vi "Dequeue.vi"() -> ()   [LabVIEW 2019]
panel:
  out "Cliente":string
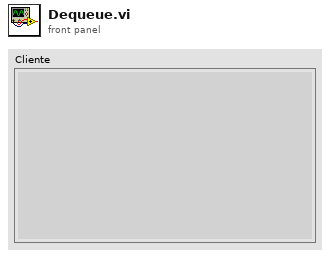
[diagram p1: front panel]
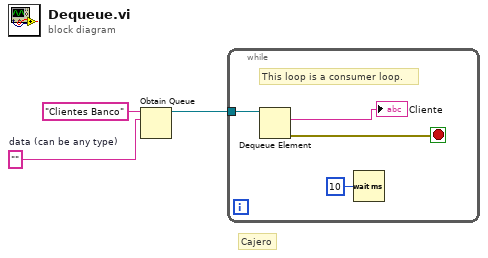
[diagram p0: block diagram]
diagram:
  w3 = ""  # data (can be any type)
  # "Cajero"
  n1 = Obtain Queue(name (unnamed)="Clientes Banco", element data type=w3) -> (queue out=w1:refnum<queue>)  [unwired: 3 in, 2 out]
  n2 = while {
    tunnel: w1 -> [w5]
    stop <- w7 stop-if-true
    # "This loop is a consumer loop."
    n3 = Dequeue Element(queue=w5) -> (element=→"Cliente":string, error out=w7:errorcluster)  [unwired: 2 in, 2 out]
    n4 = Wait (ms)(milliseconds to wait=u32 10) -> ()  [unwired: 1 out]
  }
